vi "Get SEM Results.vi"(8 "error in (no error)":errorcluster, 11 "niDTS WLAN INSTR TX in":refnum<class "niDTS WLAN INSTR TX.lvclass">) -> (0 "error out":errorcluster, 2 "SEM Results":T1, 3 "niDTS WLAN INSTR TX out":refnum<class "niDTS WLAN INSTR TX.lvclass">)   [LabVIEW 2015, in "niDTS WLAN.lvlib" / "niDTS WLAN INSTR TX.lvclass"]
uses:
  niDTS WLAN INSTR TX.lvclass
  niDTS WLAN INSTR TX INC SEM Results.ctl
  niDTS WLAN INSTR TX INC SEM FSEGemts Results.ctl
  Tests/Tx Test/Includes/Results/niDTS Tx RES INC SEM FSEGemts.ctl
  niDTS WLAN INSTR TX INC SEM MARGin Results.ctl
  Tests/Tx Test/Includes/Results/niDTS Tx RES INC SEM Margin.ctl
  niDTS WLAN INSTR TX.lvclass/niDTS WLAN INSTR TX.ctl
  RiviInstDriver/niRfsaWlan/Objects/niRfsaWlan.lvclass
  niDTS WLAN.lvlib
  RiviInstDriver/InstDriver/Objects/InstDriver.lvclass
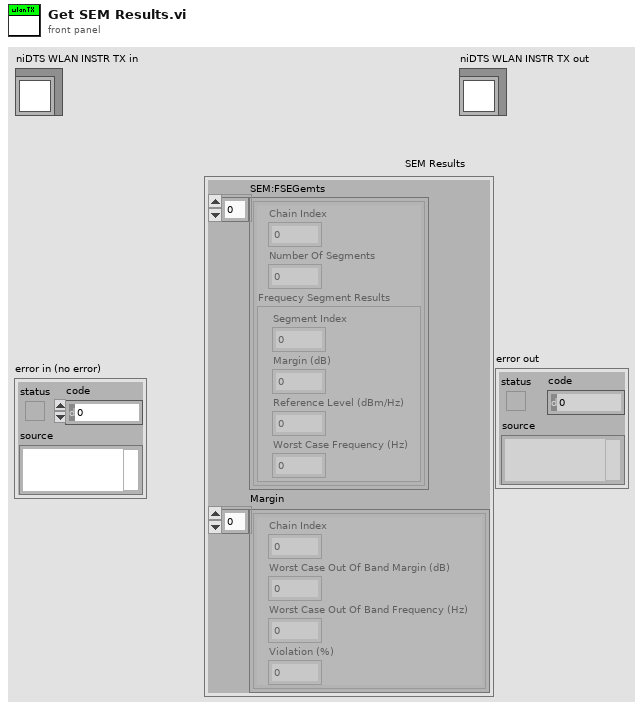
[diagram p1: front panel]
types:
  T1 = typedef "niDTS WLAN.lvlib/niDTS WLAN INSTR TX.lvclass/niDTS WLAN INSTR TX INC SEM Results.ctl" = cluster{"SEM:FSEGemts":T2, "Margin":T4}
  T2 = typedef "niDTS WLAN.lvlib/niDTS WLAN INSTR TX.lvclass/niDTS WLAN INSTR TX INC SEM FSEGemts Results.ctl" = T3[]
  T3 = typedef "niDTS WLAN.lvlib/niDTS Tx RES INC SEM FSEGemts.ctl" = cluster{"Chain Index":i32, "Number Of Segments":i32, "Frequecy Segment Results":cluster{"Segment Index":i32, "Margin (dB)":dbl, "Reference Level (dBm/Hz)":dbl, "Worst Case Frequency (Hz)":dbl}}
  T4 = typedef "niDTS WLAN.lvlib/niDTS WLAN INSTR TX.lvclass/niDTS WLAN INSTR TX INC SEM MARGin Results.ctl" = T5[]
  T5 = typedef "niDTS WLAN.lvlib/niDTS Tx RES INC SEM Margin.ctl" = cluster{"Chain Index":i32, "Worst Case Out Of Band Margin (dB)":dbl, "Worst Case Out Of Band Frequency (Hz)":dbl, "Violation (%)":dbl}
  T6 = typedef "niRfsaWlan.lvclass/niRfsaWlan INC Handle.ctl" = refnum<data-value>
  T7 = typedef "niDTS WLAN.lvlib/niDTS WLAN Tx Test INC Parameters.ctl" = cluster{"Standard":T8, "DSSS Data Rate (Mbps)":T9, "OFDM Data Rate (Mbps)":T10, "MCS Index":i32, "N spatial streams":i32, "Chains":bool[], "BandWidth (Hz)":T11, "Channel":i32, "Gard Interval":T12, "FEC Coding":T13, "Dut Tx Power":dbl, "16 symbols":bool, "payload length bytes":i32, "idle interval":dbl, "External Attenuation":dbl[], "Acquisition Parameters ":T14, "TXP Measurement Parameters":T15, "ModAcc Measurement Paramaters":T16, "ModAcc DSSS Paramaters":T17, "SEM Measurement Parameters":T19, "OBW Measurement Parameters":T20, "DSSS Power Ramp":T21, "Enable Traces":bool}
  T8 = typedef "niDTS WLAN.lvlib/niDTS WLAN INC Standard.ctl" = enum16{"802.11 b DSSS", "802.11 a/g OFDM", "802.11 n HT", "802.11 ac VHT"}
  T9 = typedef "niDTS WLAN.lvlib/niDTS WLAN INC DSSS Data Rate.ctl" = enum16{"1", "2", "5.5", "11"}
  T10 = typedef "niDTS WLAN.lvlib/niDTS WLAN INC OFDM Data Rate.ctl" = enum16{"6", "9", "12", "18", "24", "36", "48", "54"}
  T11 = typedef "niDTS WLAN.lvlib/niDTS WLAN INC CH BW.ctl" = enum16{"20 MHz", "40 MHz", "80 MHz", "160 MHz"}
  T12 = typedef "niDTS WLAN.lvlib/niDTS WLAN INC GI.ctl" = enum16{"LONG", "SHORT"}
  T13 = typedef "niDTS WLAN.lvlib/niDTS WLAN INC FEC Coding.ctl" = enum16{"BCC", "LDPC"}
  T14 = typedef "niDTS WLAN.lvlib/niDTS WLAN DUT INC Acquisition Parameters.ctl" = cluster{"Acquisition Length Mode":enum16{"AUTO", "MANUAL"}, "Acquisition Length (s)":dbl, "Auto Level":bool}
  T15 = typedef "niDTS WLAN.lvlib/niDTS WLAN INC TXP Measurement Parameters.ctl" = cluster{"TXP Power Enable":bool, "TXP Averages":i32}
  T16 = typedef "niDTS WLAN.lvlib/niDTS WLAN INC ModAcc Measurement Parameters.ctl" = cluster{"ModAcc Enable":bool, "Header Detection":enum16{"MANUAL", "FIRST", "ALL"}, "Averages":i32, "Amplitude Tracking":bool, "Channel Tracking":bool, "Time Tracking":bool, "Phase Tracking":enum16{"NONE", "STANDARD", "CSF", "INSTANT"}, "Clock Offset Est":bool, "Impairments Est":bool, "CFO Estimation":enum16{"PAMBLE", "PDATA"}}
  T17 = typedef "niDTS WLAN.lvlib/niDTS WLAN INC DSSS ModAcc Measurement Parameters.ctl" = cluster{"DC Offset Compensation":bool, "Equalization":bool, "Phase Tracking":bool, "Chip Start Location":i16, "Max Chips Used":i16, "Pulse Shaping FilterType":T18, "Pulse Shaping Filter Coefficient":dbl}
  T18 = typedef "niDTS WLAN.lvlib/niDTS WLAN INC Pulse Shaping Filter Type.ctl" = enum16{"NONE", "RCOSINE", "RRCOSINE", "GAUSSIAN"}
  T19 = typedef "niDTS WLAN.lvlib/niDTS WLAN INC SEM Measurement Parameters.ctl" = cluster{"SEM Enable":bool, "SEM Averages":i32, "Auto Span Enable":bool, "Frequency Span (Hz)":dbl, "Measurement Type":enum16{"Standard", "Legacy", "Custom"}, "Mask Frequencies (Hz)":dbl[], "Mask Power Offsets (dB)":dbl[]}
  T20 = typedef "niDTS WLAN.lvlib/niDTS WLAN INC OBW Measurement Parameters.ctl" = cluster{"OBW Enable":bool, "OBW Averages":i32}
  T21 = typedef "niDTS WLAN.lvlib/niDTS WLAN INC DSSS Power Ramp Parameters.ctl" = cluster{"Power Ramp Enable":bool, "Averages":i32, "Thresholds":cluster{"Up Low (%)":dbl, "Down Low (%)":dbl, "Up High (%)":dbl, "Down High (%)":dbl}}
  T22 = cluster{"ChainIndex":i32, "WorstCaseOutOfBandMargin":dbl, "WorstCaseOutOfBandFrequency":dbl, "Violation":dbl}[]
  T23 = typedef "InstDriver.lvclass/niInstDriver INC Handle.ctl" = refnum<data-value>
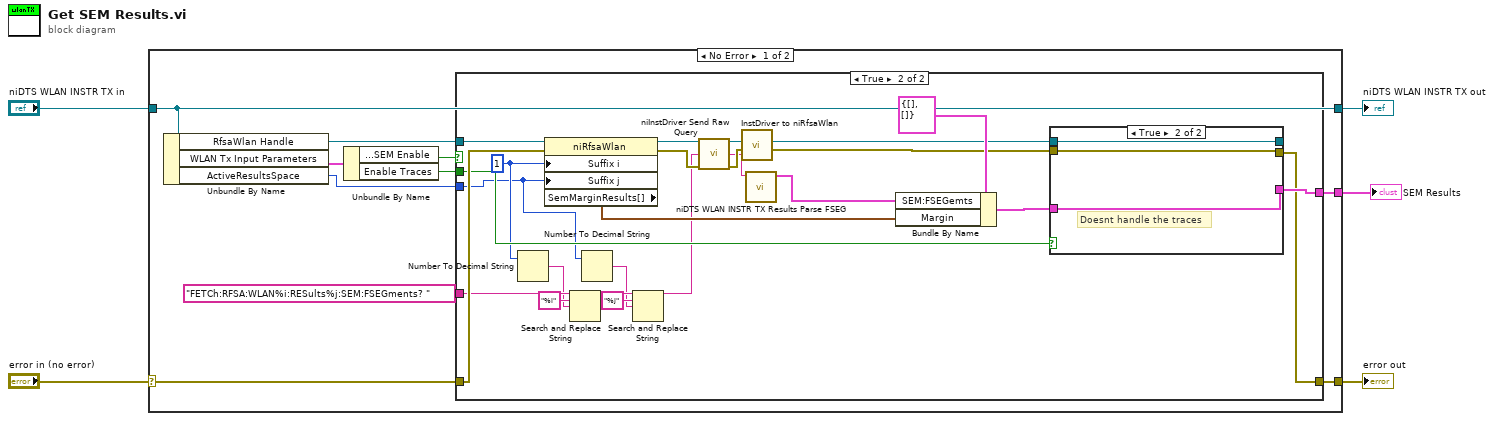
[diagram p0: block diagram]
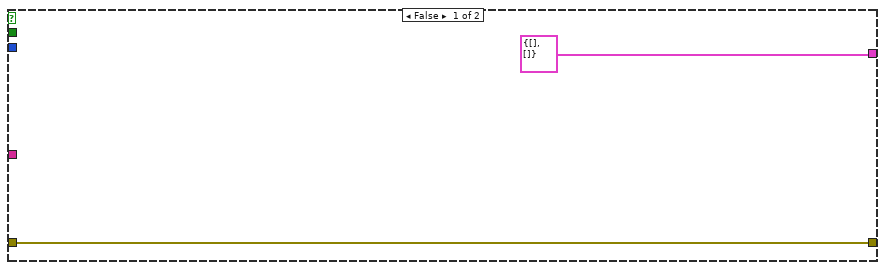
[diagram p2: hidden frame]
diagram:
  n1 = case shown="No Error" "error in (no error)" {
    selector: "error in (no error)" -> [w13 w50]
    tunnel: [w9 w50] -> w4
    tunnel: [w15 w49] -> w2
    tunnel: "niDTS WLAN INSTR TX in" -> [w15 w49]
    tunnel: [w10 _] -> w1
    frame No Error {
      n2 = Unbundle By Name(w15) -> ("RfsaWlan Handle"=w11:T6, "WLAN Tx Input Parameters"=w14:T7, "ActiveResultsSpace"=w7:u8)
      n3 = Unbundle By Name(w14) -> ("SEM Measurement Parameters.SEM Enable"=w12:bool, "Enable Traces"=w8:bool)
      n4 = case shown="True" w12 {
        tunnel: w13 -> [w17 w40]
        tunnel: w11 -> [_ w42]
        tunnel: [T1 {"SEM:FSEGemts"=[], "Margin"=[]} ("SEM Results") w41] -> w10
        tunnel: [w17 w39] -> w9
        tunnel: w8 -> [_ w38]
        tunnel: w7 -> [_ w22]
        tunnel: "FETCh:RFSA:WLAN%i:RESults%j:SEM:FSEGments? " -> [_ w28]
        frame False {
        }
        frame True {
          w24 = 1 ("Active Channel:Suffix i")
          n5 = Number To Decimal String(number=w24) -> (decimal integer string=w23:string)  [unwired: 1 in]
          n6 = property class="niRfsaWlan"(reference=w42, error in=w40, "Suffix i"=w24, "Suffix j"=w22) -> (reference out=w32:T6, error out=w31:errorcluster, "SemMarginResults[]"=w35:T22)
          n7 = Search and Replace String(input string=w28, search string="%i", replace string=w23) -> (result string=w26:string)  [unwired: 5 in, 3 out]
          n8 = Number To Decimal String(number=w22) -> (decimal integer string=w21:string)  [unwired: 1 in]
          n9 = Search and Replace String(input string=w26, search string="%j", replace string=w21) -> (result string=w20:string)  [unwired: 5 in, 3 out]
          n10 = call "niInstDriver Send Raw Query.vi"("InstDriver Handle in"=w32, "Query"=w20, "error in (no error)"=w31) -> ("InstDriver Handle out"=w34:T23, "Response"=w19:string, "error out"=w33:errorcluster)  [unwired: 10 in]
          n11 = call "InstDriver to niRfsaWlan.vi"("error in (no error)"=w33, "InstDriver Handle in"=w34) -> ("error out"=w30:errorcluster, "InstDriver Handle out"=w29:refnum<data-value>)  [unwired: 8 in]
          n12 = call "niDTS WLAN INSTR TX Results Parse FSEG.vi"("String"=w19) -> ("SEM:FSEGemts"=w18:T2)  [unwired: 10 in]
          n13 = Bundle By Name(cluster=T1 {"SEM:FSEGemts"=[], "Margin"=[]} ("SEM Results"), "SEM:FSEGemts"=w18, "Margin"=w35) -> (w36:T1)
          n14 = case shown="True" w38 {
            tunnel: w29 -> [w43 w47]
            tunnel: w30 -> [w45 w46]
            tunnel: w36 -> [w44 w48]
            tunnel: [w45 w46] -> w39
            tunnel: [w44 w48] -> w41
            tunnel: [w43 w47] -> _
            frame False {
            }
            frame True {
              # "Doesnt handle the traces"
            }
          }
        }
      }
    }
    frame Error {
    }
  }
  "error out" <- w4
  "niDTS WLAN INSTR TX out" <- w2
  "SEM Results" <- w1
